vi "Test - Extract Sequence Parameters.vi"(8 "error in (no error)":errorcluster, 10 "Sequence Data":string[][](array[string]), 11 "Cluster in":T1={"Preslip Sequence"=[], "Step No"=0, "Step Value"={"Sr.no"=0, "Log?"=FALSE, "Step"="", "Type"="", "Channel"="", "Value"=0.0, "Para1"=0.0, "Para2"=0.0, "Limit1"=0.0, "Limit2"=0.0, "Comparision Mode"="", "Timeout"=0.0}, "Slip Parameter"=[], "Slip Timer"=0.0, "Postslip Sequence"=[], "Postslip ?"=FALSE, "Step Result"={"Step Name"="", "Value"=0.0, "Success ?"=TRUE, "Stop Seq ?"=TRUE, "Abort"=TRUE, "Sr.No"=0}}) -> (0 "error out":errorcluster, 3 "output cluster":T1={"Preslip Sequence"=[], "Step No"=0, "Step Value"={"Sr.no"=0, "Log?"=FALSE, "Step"="", "Type"="", "Channel"="", "Value"=0.0, "Para1"=0.0, "Para2"=0.0, "Limit1"=0.0, "Limit2"=0.0, "Comparision Mode"="", "Timeout"=0.0}, "Slip Parameter"=[], "Slip Timer"=0.0, "Postslip Sequence"=[], "Postslip ?"=FALSE, "Step Result"={"Step Name"="", "Value"=0.0, "Success ?"=TRUE, "Stop Seq ?"=TRUE, "Abort"=TRUE, "Sr.No"=0}})   [LabVIEW 2017]
uses:
  Test - Message cluster.ctl
  Test - Step config.ctl
  Test - Step Result.ctl
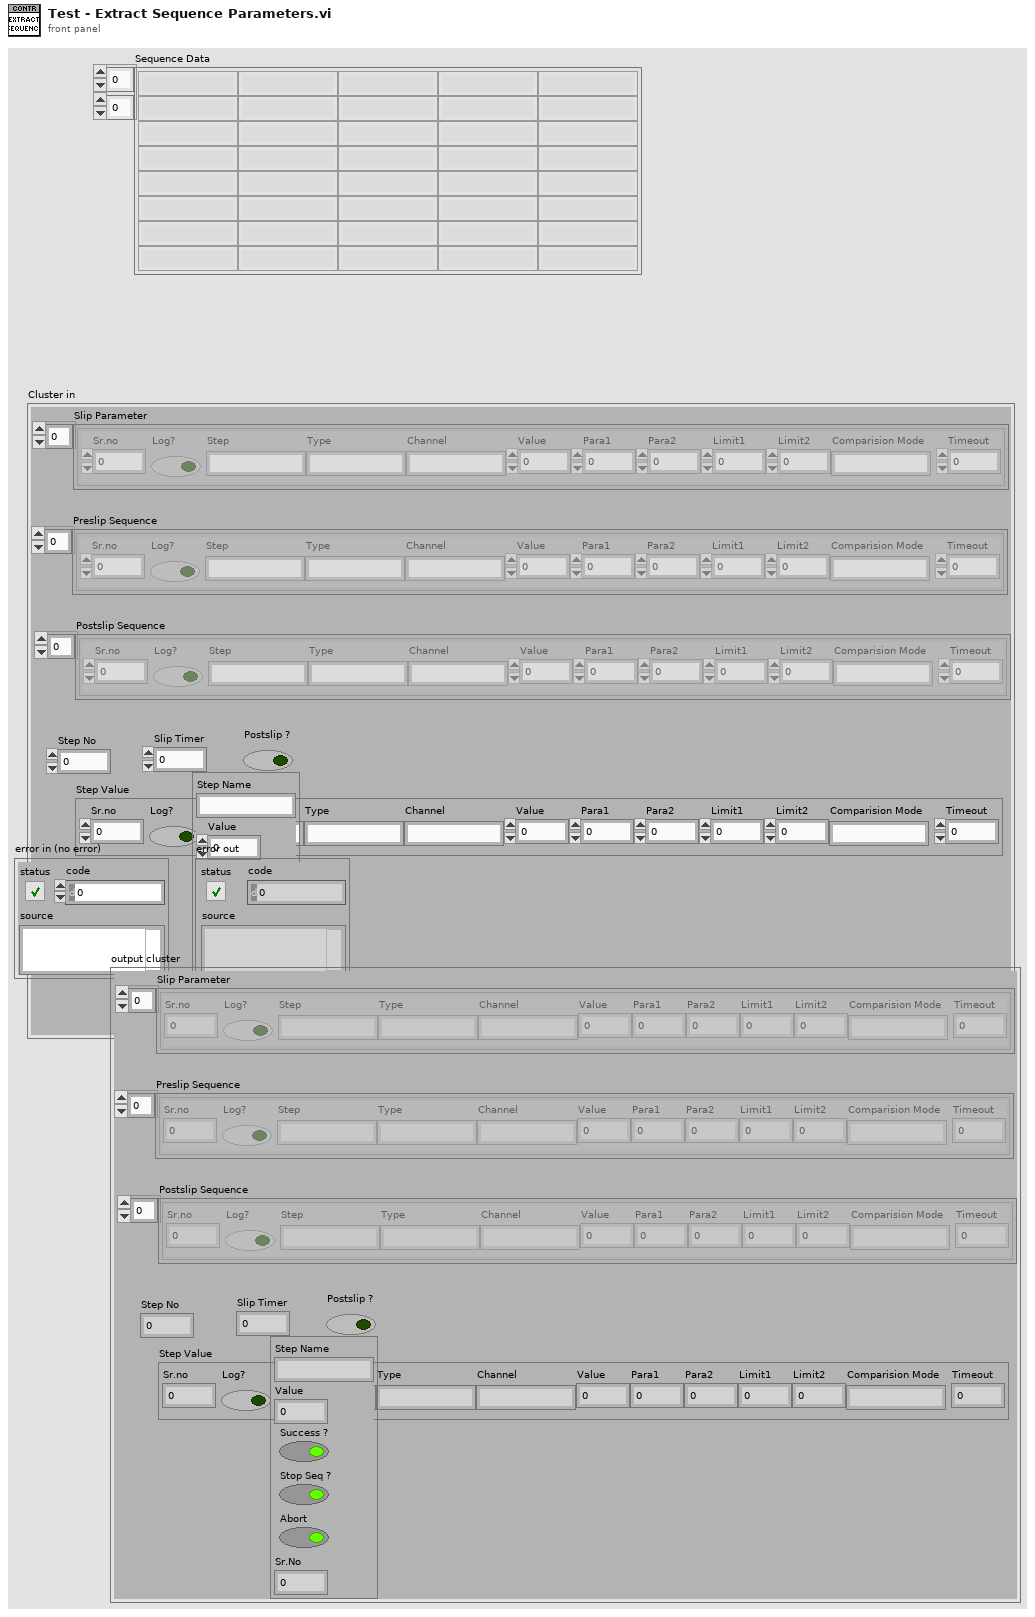
[diagram p1: front panel]
types:
  T1 = typedef "Test - Message cluster.ctl" = cluster{"Preslip Sequence":T2[], "Step No":i32, "Step Value":T2, "Slip Parameter":T2[], "Slip Timer":dbl, "Postslip Sequence":T2[], "Postslip ?":bool, "Step Result":T3}
  T2 = typedef "Test - Step config.ctl" = cluster{"Sr.no":i32, "Log?":bool, "Step":string, "Type":string, "Channel":string, "Value":dbl, "Para1":dbl, "Para2":dbl, "Limit1":dbl, "Limit2":dbl, "Comparision Mode":string, "Timeout":dbl}
  T3 = typedef "Test - Step Result.ctl" = cluster{"Step Name":string, "Value":dbl, "Success ?":bool, "Stop Seq ?":bool, "Abort":bool, "Sr.No":i32}
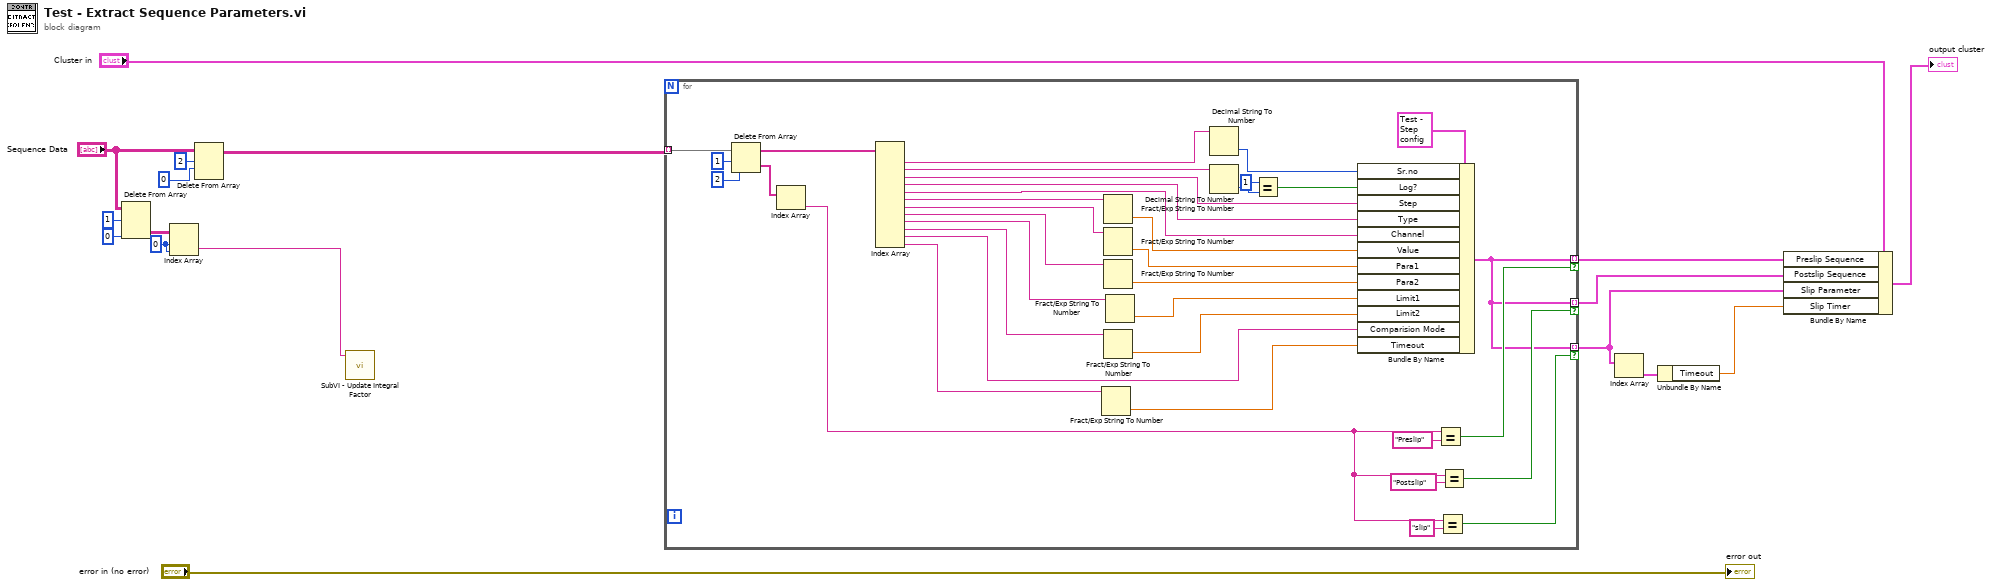
[diagram p0: block diagram]
diagram:
  w3 = 0 ("index (row)")
  n1 = Delete From Array(array="Sequence Data", length=1, index (row)=0) -> (deleted portion=w4:string[][])  [unwired: 1 in, 1 out]
  n2 = Index Array(array=w4, index (row)=w3, index (col)=w3) -> (element=w2:string)
  n3 = Delete From Array(array="Sequence Data", length=2, index (row)=0) -> (array with subset deleted=w13:string[][])  [unwired: 1 in, 1 out]
  n4 = call "SubVI - Update Integral Factor.vi"("Delta Torque"=w2) -> ()  [unwired: 11 in]
  n5 = for {
    tunnel: w13 -> [w27] mode=indexing
    tunnel: [w20] -> w15 mode=indexing if=w25
    tunnel: [w20] -> w10 mode=indexing if=w23
    tunnel: [w20] -> w9 mode=indexing if=w19
    n6 = Delete From Array(array=w27, length=1, index=2 ("index (row)")) -> (deleted portion=w29:string[], array with subset deleted=w26:string[])
    n7 = Index Array(array=w29) -> (element=w21:string)  [unwired: 1 in]
    n8 = Index Array(array=w26) -> (element #1=w52:string, element #2=w51:string, element #3=w48:string, element #4=w47:string, element #5=w46:string, element #6=w45:string, element #7=w43:string, element #8=w41:string, element #9=w39:string, element #10=w37:string, element #11=w35:string, element #12=w34:string)  [unwired: 12 in]
    n9 = Fract/Exp String To Number(string=w34) -> (number=w33:dbl)  [unwired: 3 in, 1 out]
    n10 = Fract/Exp String To Number(string=w45) -> (number=w44:dbl)  [unwired: 3 in, 1 out]
    n11 = Fract/Exp String To Number(string=w43) -> (number=w42:dbl)  [unwired: 3 in, 1 out]
    n12 = Fract/Exp String To Number(string=w41) -> (number=w40:dbl)  [unwired: 3 in, 1 out]
    n13 = Fract/Exp String To Number(string=w37) -> (number=w36:dbl)  [unwired: 3 in, 1 out]
    n14 = Fract/Exp String To Number(string=w39) -> (number=w38:dbl)  [unwired: 3 in, 1 out]
    n15 = Decimal String To Number(string=w52) -> (number=w53:i32)  [unwired: 2 in, 1 out]
    n16 = Decimal String To Number(string=w51) -> (number=w50:i32)  [unwired: 2 in, 1 out]
    n17 = Equal?(x=1, y=w50) -> (x = y?=w49:bool)
    n18 = Bundle By Name(cluster=T2 {"Sr.no"=0, "Log?"=FALSE, "Step"="", "Type"="", "Channel"="", "Value"=0.0, "Para1"=0.0, "Para2"=0.0, "Limit1"=0.0, "Limit2"=0.0, "Comparision Mode"="", "Timeout"=0.0} ("Cluster"), "Sr.no"=w53, "Log?"=w49, "Step"=w48, "Type"=w47, "Channel"=w46, "Value"=w44, "Para1"=w42, "Para2"=w40, "Limit1"=w38, "Limit2"=w36, "Comparision Mode"=w35, "Timeout"=w33) -> (w20:T2)
    n19 = Equal?(x=w21, y="Preslip") -> (x = y?=w25:bool)
    n20 = Equal?(x=w21, y="slip") -> (x = y?=w19:bool)
    n21 = Equal?(x=w21, y="Postslip") -> (x = y?=w23:bool)
  }
  n22 = Index Array(array=w9) -> (element=w8:T2)  [unwired: 1 in]
  n23 = Unbundle By Name(w8) -> ("Timeout"=w7:dbl)
  n24 = Bundle By Name(cluster="Cluster in", "Preslip Sequence"=w15, "Postslip Sequence"=w10, "Slip Parameter"=w9, "Slip Timer"=w7) -> (→"output cluster":T1)
  "error out" <- "error in (no error)"
